vi "Unpack Message.vi"(8 "error in (no error)":errorcluster, 9 "Packed Message":string, 10 "Message Name":string, 11 "Message String in":refnum<class "Message String.lvclass">) -> (0 "error out":errorcluster, 2 "Valid":bool, 3 "Message String out":refnum<class "Message String.lvclass">)   [LabVIEW 2016, in "Stream Mediator.lvlib" / "Message String.lvclass"]
uses:
  <userlib>/Composed Systems/Stream/Mediator/Classes/Message String/Message String.lvclass
  C:/Program Files (x86)/National Instruments/LabVIEW 2016/user.lib/Composed Systems/Stream/Mediator/Classes/Message Interface/Message Interface.lvclass
  <userlib>/Composed Systems/Stream/Mediator/Classes/Message String/Message String.lvclass/Message String.ctl
  <userlib>/Composed Systems/Stream/Mediator/Classes/Message Interface/Message Interface.lvclass
  <vilib>/addons/_JKI.lib/Serialization/JSON/JKI JSON Serialization.lvlib
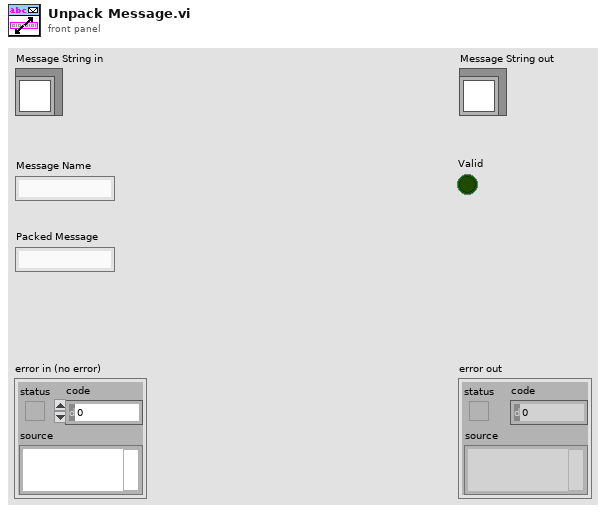
[diagram p1: front panel]
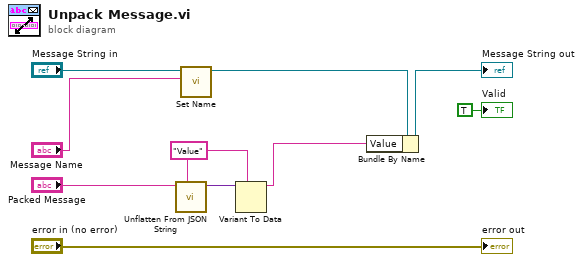
[diagram p0: block diagram]
diagram:
  w3 = "Value"
  n1 = call <vilib>:"Unflatten From JSON String.vi"("Type and Defaults"=w3, "JSON String"="Packed Message") -> ("Variant"=w4:variant)  [unwired: 8 in, 1 out]
  n2 = call <userlib>:"Set Name.vi"("Name"="Message Name", "Message Interface in"="Message String in") -> ("Message Interface out"=w10:refnum<class "Message String.lvclass">)  [unwired: 8 in, 1 out]
  n3 = Variant To Data(type=w3, Variant=w4) -> (data=w2:string)  [unwired: 1 in, 1 out]
  n4 = Bundle By Name(cluster=w10, "Value"=w2) -> (→"Message String out":refnum<class "Message String.lvclass">)
  "error out" <- "error in (no error)"
  "Valid" <- TRUE ("Valid")
